vi "set_config_cluster.vi"(8 "error in (no error)":errorcluster, 10 "config cluster variant":variant, 11 "InstrumentDL090324 in":refnum<class "InstrumentDL090324.lvclass">) -> (0 "error out":errorcluster, 3 "InstrumentDL090324 out":refnum<class "InstrumentDL090324.lvclass">)   [LabVIEW 2010, in "InstrumentDL090324.lvclass"]
uses:
  InstrumentDL090324.lvclass
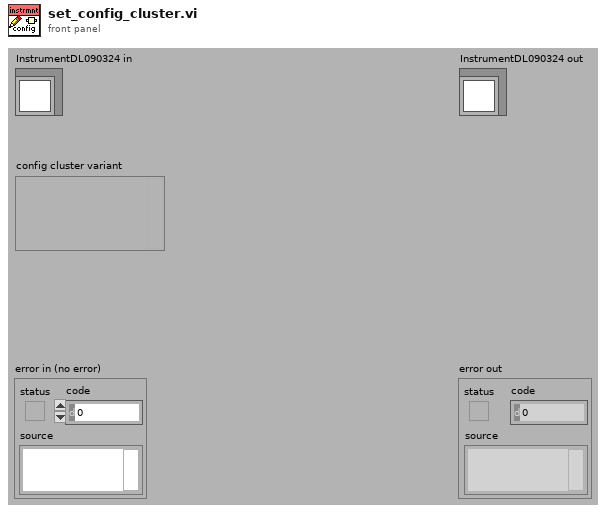
[diagram p1: front panel]
types:
  T1 = typedef "InstrumentDL090324.lvclass/config_data_cluster.ctl" = cluster{"detectors":T2[], "LSID":T3, "light source":T2[]}
  T2 = typedef "plugin_specification.ctl" = cluster{"class path":string, "configuration":string, "label":string, "settings name":string}
  T3 = typedef "LSID_cluster.ctl" = cluster{"identifier":string, "revision":i32}
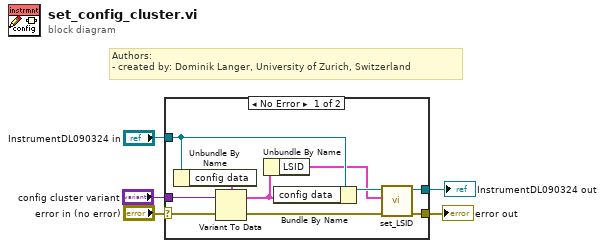
[diagram p0: block diagram]
diagram:
  # "Authors: \n- created by: Dominik Langer, University of Zurich, Switzerland"
  n1 = case shown="No Error" "error in (no error)" {
    selector: "error in (no error)" -> [w14 w16]
    tunnel: [w6 w16] -> w2
    tunnel: "InstrumentDL090324 in" -> [w8 w17]
    tunnel: [w10 w17] -> w1
    tunnel: "config cluster variant" -> [w12 _]
    frame No Error {
      n2 = Unbundle By Name(w8) -> ("config data"=w13:T1)
      n3 = Variant To Data(error in=w14, Variant=w12, type=w13) -> (error out=w15:errorcluster, data=w11:cluster{})
      n4 = Unbundle By Name(w11) -> ("LSID"=w7:T3)
      n5 = Bundle By Name(cluster=w8, "config data"=w11) -> (w9:refnum<class "InstrumentDL090324.lvclass">)
      n6 = call-dynamic "set_LSID.vi"("error in (no error)"=w15, "LSID"=w7, "GenericPlugin in"=w9) -> ("error out"=w6:errorcluster, "GenericPlugin out"=w10:refnum<class "InstrumentDL090324.lvclass">)  [unwired: 7 in]
    }
    frame Error {
    }
  }
  "error out" <- w2
  "InstrumentDL090324 out" <- w1
